vi "Lock Controls.vi"(8 "error in (no error)":errorcluster, 10 "Lock Controls?":bool, 11 "DPO4104 in":refnum<class "DPO4104.lvclass">) -> (0 "error out":errorcluster, 3 "DPO4104 out":refnum<class "DPO4104.lvclass">)   [LabVIEW 2018, in "DPO4104.lvlib" / "DPO4104.lvclass"]
doc: "This override method is used to lock/unlock user access to the oscilloscope front panel controls."
uses:
  DPO4104.lvclass
  PPLs/Oscilloscope/Parent/Oscilloscope.lvlibp/Oscilloscope.lvclass
  C:/Projects/LabVIEW/PPLs/Oscilloscope/Parent/Oscilloscope.lvlibp/Oscilloscope.lvclass
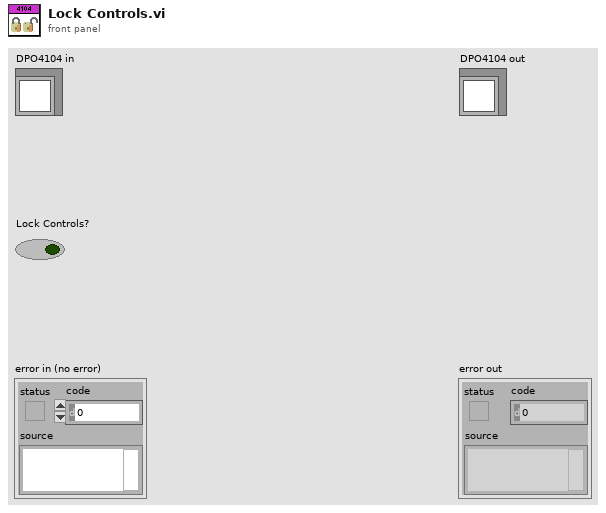
[diagram p1: front panel]
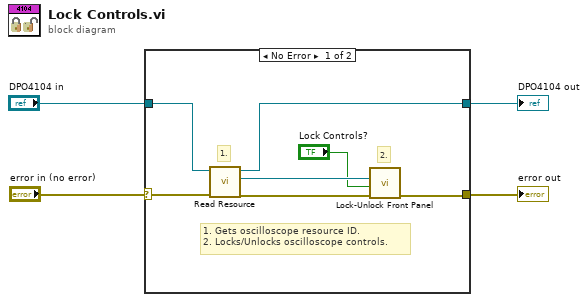
[diagram p0: block diagram]
diagram:
  n1 = case shown="No Error" "error in (no error)" {
    selector: "error in (no error)" -> [w6 w12]
    tunnel: [w7 w12] -> w3
    tunnel: "DPO4104 in" -> [w11 w13]
    tunnel: [w10 w13] -> w1
    frame No Error {
      # "1. Gets oscilloscope resource ID.\n2. Locks/Unlocks oscilloscope controls."
      # "2."
      # "1."
      n2 = call "Read Resource.vi"("error in (no error)"=w6, "Oscilloscope in"=w11) -> ("error out"=w8:errorcluster, "Resource"=w9:refnum<visa-resource-name>, "Oscilloscope out"=w10:refnum<class "DPO4104.lvclass">)  [unwired: 7 in]
      n3 = call "Lock-Unlock Front Panel.vi"("error in (no error)"=w8, "Lock?"="Lock Controls?", "VISA resource name"=w9) -> ("error out"=w7:errorcluster)  [unwired: 6 in, 2 out]
    }
    frame Error {
    }
  }
  "error out" <- w3
  "DPO4104 out" <- w1
